vi "Test 2 Inflate Universe.vi"(8 "error in (no error)":errorcluster, 11 "Test Case In":refnum<class "Day X Test.lvclass">) -> (0 "error out":errorcluster, 3 "Test Case Out":refnum<class "Day X Test.lvclass">)   [LabVIEW 2020, in "Day X Test.lvclass"]
uses:
  Day X Test.lvclass
  C:/Program Files (x86)/National Instruments/LabVIEW 2020/vi.lib/Astemes/LUnit/Test Case.lvclass
  <vilib>/Astemes/LUnit/Test Case.lvclass/Test Case.ctl
  4993e8ee-a06a-463a-9684-69129f64d5ce.vi
  <vilib>/Astemes/LUnit/Append Pass Result.vi
  <vilib>/Astemes/LUnit/Append Fail Result.vi
  <vilib>/Astemes/LUnit/Describe Comparison.vi
  <vilib>/Astemes/LUnit/Compare Variants.vi
  <vilib>/Astemes/LUnit/Variant to string.vi
  <vilib>/Utility/Data Type/Get Type Information.vi
  <vilib>/Utility/LVClass/Get LV Class Name.vi
  Day X Test.lvclass/Day X Test.ctl
  Galaxy/Galaxy.lvclass
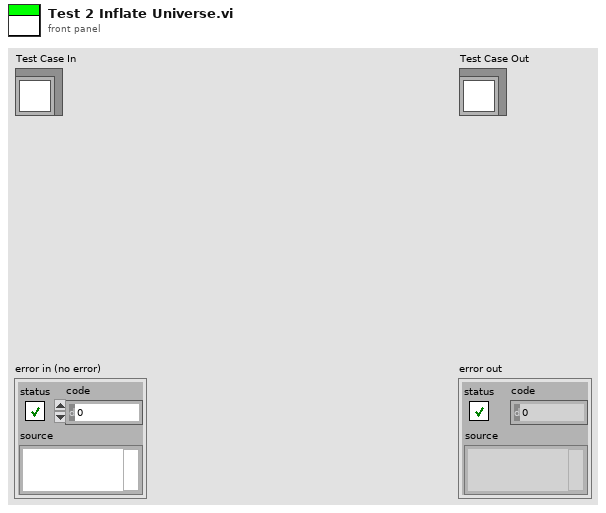
[diagram p1: front panel]
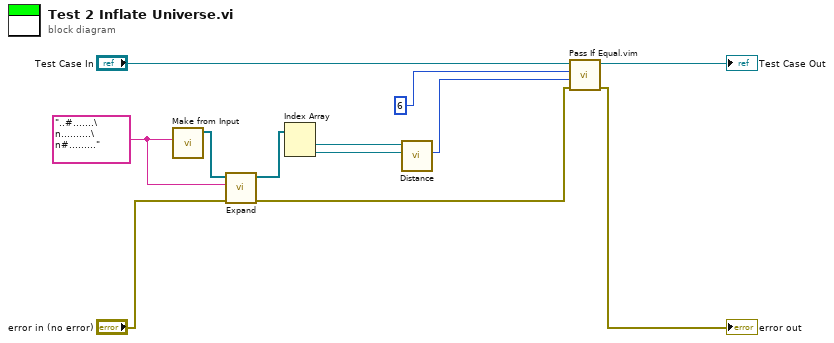
[diagram p0: block diagram]
diagram:
  w2 = "..#.......\n..........\n#........."
  n1 = call "Make from Input.vi"("Input"=w2) -> ("Galaxy out"=w9:refnum<class "Galaxy.lvclass">[])  [unwired: 9 in, 1 out]
  n2 = call "Expand.vi"("error in (no error)"="error in (no error)", "Input"=w2, "Galaxy in"=w9) -> ("error out"=w3:errorcluster, "Array"=w4:refnum<class "Galaxy.lvclass">[])  [unwired: 7 in]
  n3 = Index Array(array=w4) -> (element #1=w8:refnum<class "Galaxy.lvclass">, element #2=w7:refnum<class "Galaxy.lvclass">)  [unwired: 2 in]
  n4 = call "Distance.vi"("Galaxy in 2"=w7, "Galaxy in"=w8) -> ("Numeric"=w6:u64)  [unwired: 8 in, 1 out]
  n5 = call "Pass If Equal.vim"("error in (no error)"=w3, "Actual"=w6, "Expected"=u64 6 ("Numeric"), "LUnit Test Case In"="Test Case In") -> ("error out"=→"error out":errorcluster, "LUnit Test Case Out"=→"Test Case Out":refnum<class "Day X Test.lvclass">)  [unwired: 6 in]
